vi "manage relay LED colors.vi"(0 "RelayValue":T2, 11 "RelayDirection":T1) -> (8 "LED color":u32(colorbox)=1985280)   [LabVIEW 2025]
doc: "This subVI controls the LED color to match that of the SPIKE relay."
uses:
  <vilib>/Rock Robotics/WPI/Relay/WPI_RelayValue.ctl
  <vilib>/Rock Robotics/WPI/Relay/WPI_RelayDirection.ctl
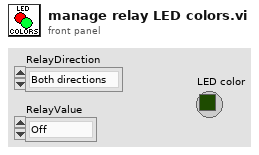
[diagram p1: front panel]
types:
  T1 = typedef "WPI_RelayDirection.ctl" = enum16{"Both directions", "Forward only", "Reverse only"}
  T2 = typedef "WPI_RelayValue.ctl" = enum16{"Off", "On", "Forward", "Reverse"}
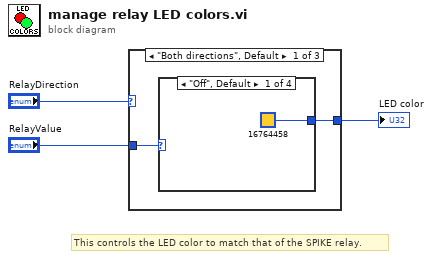
[diagram p0: block diagram]
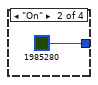
[diagram p2: hidden frame]
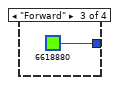
[diagram p3: hidden frame]
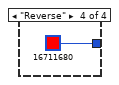
[diagram p4: hidden frame]
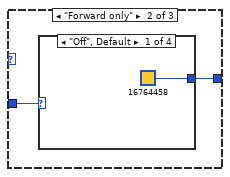
[diagram p5: hidden frame]
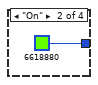
[diagram p6: hidden frame]
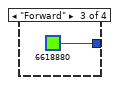
[diagram p7: hidden frame]
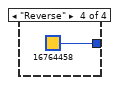
[diagram p8: hidden frame]
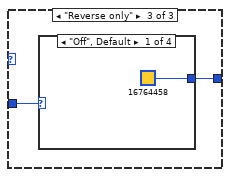
[diagram p9: hidden frame]
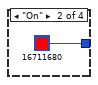
[diagram p10: hidden frame]
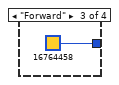
[diagram p11: hidden frame]
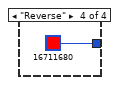
[diagram p12: hidden frame]
diagram:
  # "This controls the LED color to match that of the SPIKE relay."
  n1 = case shown="\"Both directions\", Default" "RelayDirection" {
    tunnel: "RelayValue" -> [w5 w11 w17]
    tunnel: [w4 w10 w16] -> w1
    frame "Both directions", Default {
      n2 = case shown="\"Off\", Default" w5 {
        tunnel: [u32 16764458 ("Color Box") u32 1985280 ("Color Box") u32 6618880 ("Color Box") u32 16711680 ("Color Box")] -> w4
        frame "Off", Default {
        }
        frame "On" {
        }
        frame "Forward" {
        }
        frame "Reverse" {
        }
      }
    }
    frame "Forward only" {
      n3 = case shown="\"Off\", Default" w11 {
        tunnel: [u32 16764458 ("Color Box") u32 6618880 ("Color Box") u32 6618880 ("Color Box") u32 16764458 ("Color Box")] -> w10
        frame "Off", Default {
        }
        frame "On" {
        }
        frame "Forward" {
        }
        frame "Reverse" {
        }
      }
    }
    frame "Reverse only" {
      n4 = case shown="\"Off\", Default" w17 {
        tunnel: [u32 16764458 ("Color Box") u32 16711680 ("Color Box") u32 16764458 ("Color Box") u32 16711680 ("Color Box")] -> w16
        frame "Off", Default {
        }
        frame "On" {
        }
        frame "Forward" {
        }
        frame "Reverse" {
        }
      }
    }
  }
  "LED color" <- w1
